vi "数据库查询.vi"() -> ()   [LabVIEW 2018]
uses:
  <vilib>/addons/_office/_exclsub.llb/font.ctl
  <vilib>/addons/database/Connection.llb/DB Tools Open Connec (String).vi
  <vilib>/addons/_office/excel.llb/Excel Easy Table (str).vi
  <vilib>/Utility/NIReport.llb/NI_report.lvclass
  <vilib>/addons/database/NI_Database_API.lvlib
  <vilib>/addons/_office/NI_ReportGenerationToolkit.lvlib
  <vilib>/Utility/NIReport.llb/Excel/NI_Excel.lvclass
panel:
  in  "Main Tab":enum32{""}(tab)
  in  "时间范围OFF":bool
  out "查询状态":string
  in  "总成码OFF":bool
  in  "刻印码":string
  in  "导出":bool
  in  "退出":bool
  in  "查询结果":i32(listbox)
  in  "查询":bool
  in  "另存为":bool
  in  "二维码OFF":bool
  in  "二维码":string
  in  "结束日期":timestamp
  in  "起始日期":timestamp
  in  "数据类型":u16(ring) items=["ALL", "Online", "Offline", "Rework"]
  in  "产品状态":u16(ring) items=["ALL", "OK", "NG"]
  # "历史数据查询"
  # "期间（过滤器）"
  # "运行"
  # "驱动数据（过滤器）"
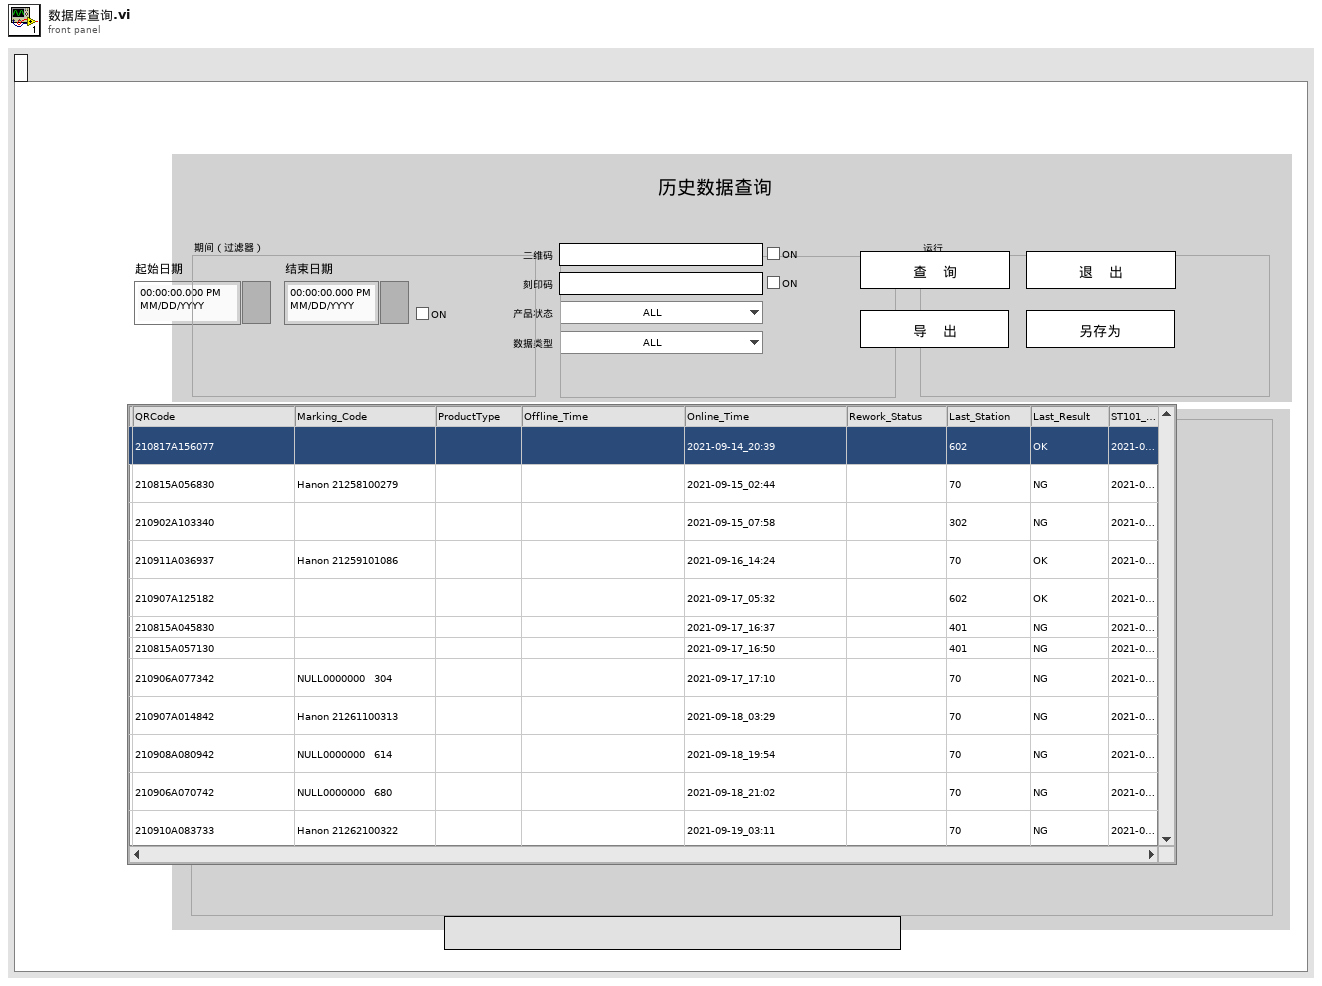
[diagram p1: front panel]
types:
  T1 = typedef "NI_ReportGenerationToolkit.lvlib/font.ctl" = cluster{"font name":string, "font size":dbl, "bold":u16, "italic":u16, "underline":u16, "strike through":u16, "font color":u32}
  T2 = enum16{"Standard Report", "HTML", "Word", "Excel"}
  T3 = enum16{"maximized", "minimized", "normal", "no change"}
  T4 = enum32{"Invalid", "Standard", "Closed", "Hidden", "Minimized", "Maximized"}
  T5 = typedef "NI_Database_API.lvlib/Conn ObjectReference.ctl" = refnum<k1>
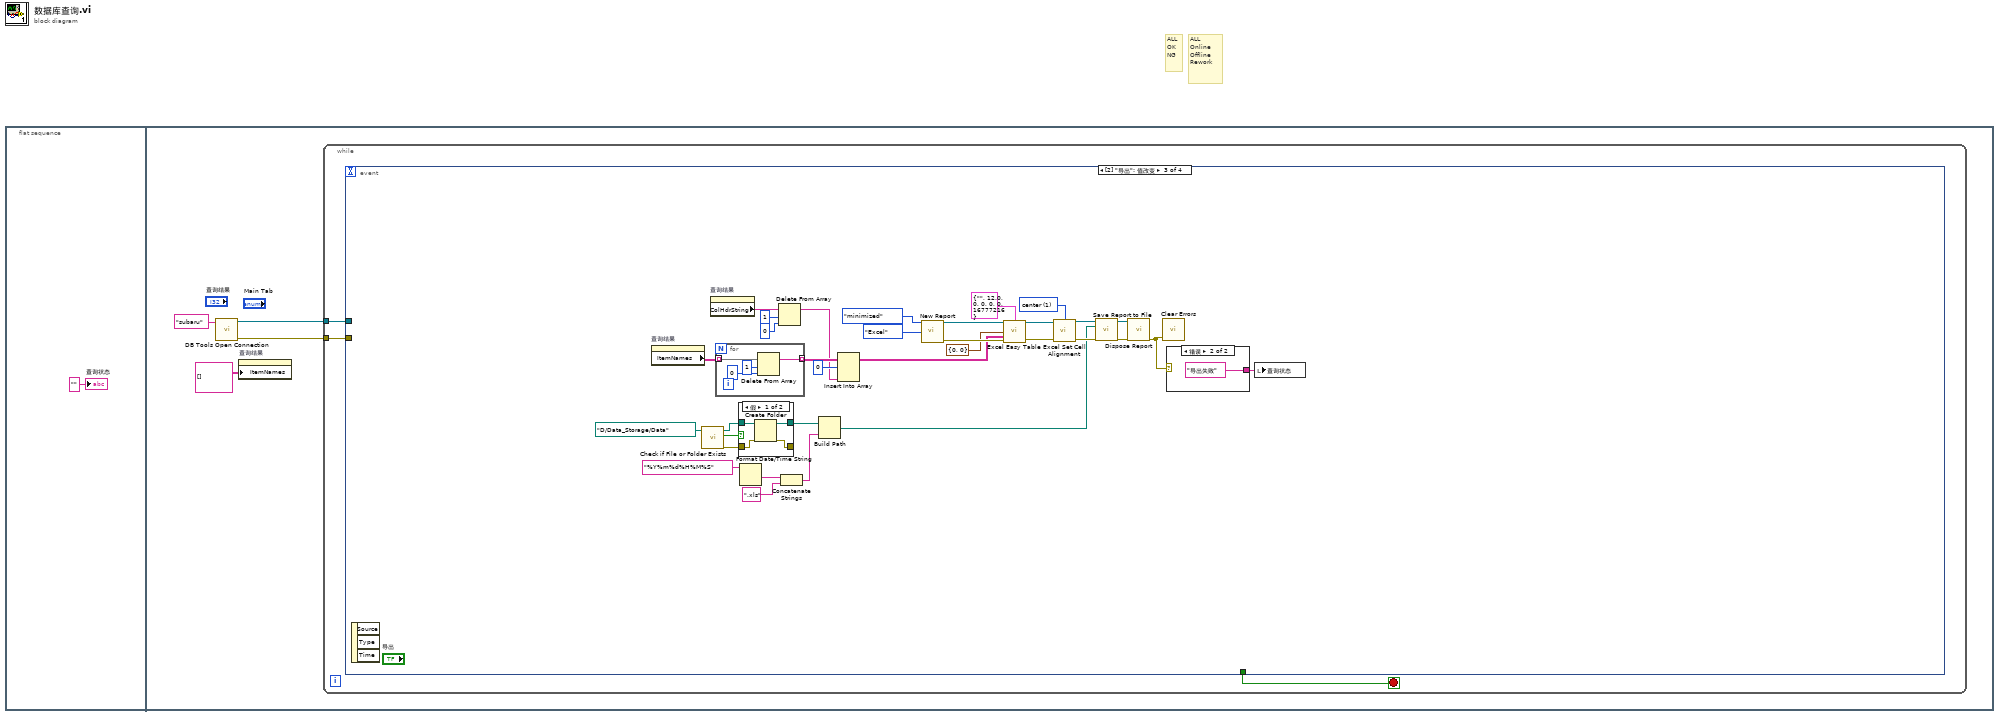
[diagram p0: block diagram]
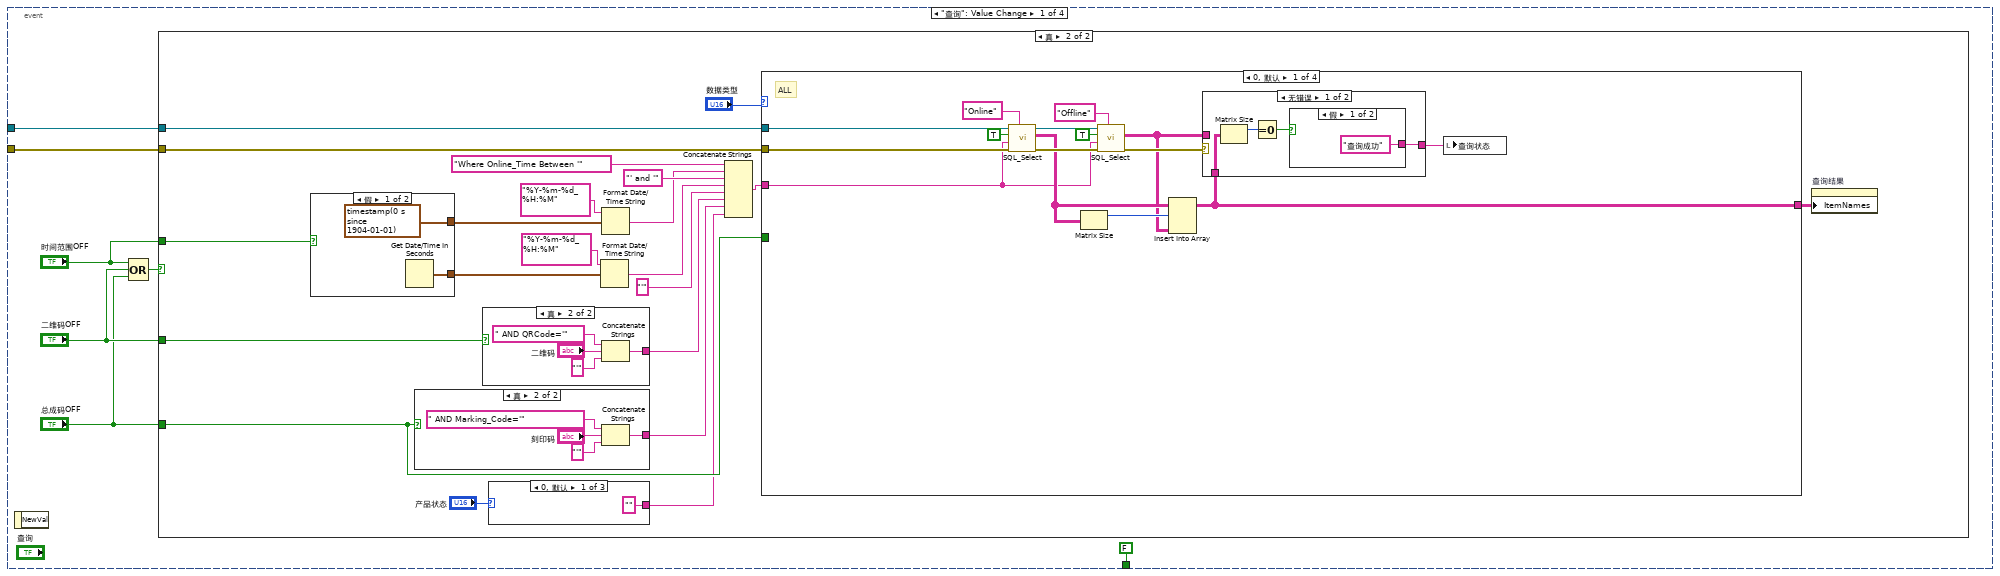
[diagram p2: hidden frame]
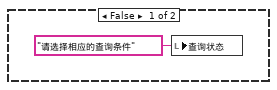
[diagram p3: hidden frame]
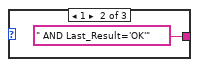
[diagram p4: hidden frame]
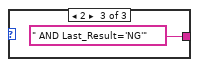
[diagram p5: hidden frame]
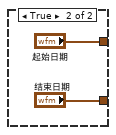
[diagram p6: hidden frame]
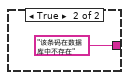
[diagram p7: hidden frame]
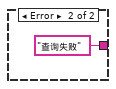
[diagram p8: hidden frame]
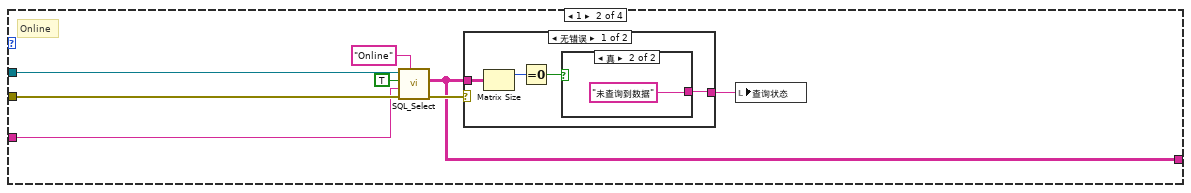
[diagram p9: hidden frame]
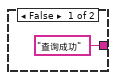
[diagram p10: hidden frame]
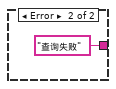
[diagram p11: hidden frame]
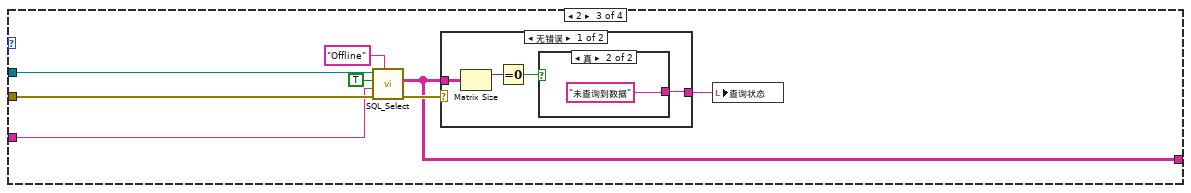
[diagram p12: hidden frame]
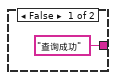
[diagram p13: hidden frame]
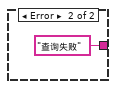
[diagram p14: hidden frame]
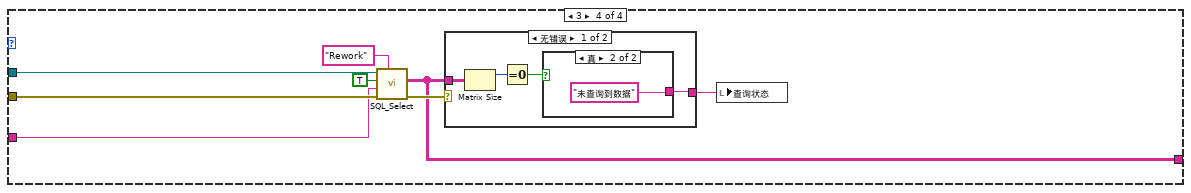
[diagram p15: hidden frame]
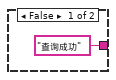
[diagram p16: hidden frame]
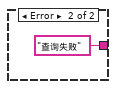
[diagram p17: hidden frame]
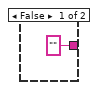
[diagram p18: hidden frame]
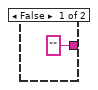
[diagram p19: hidden frame]
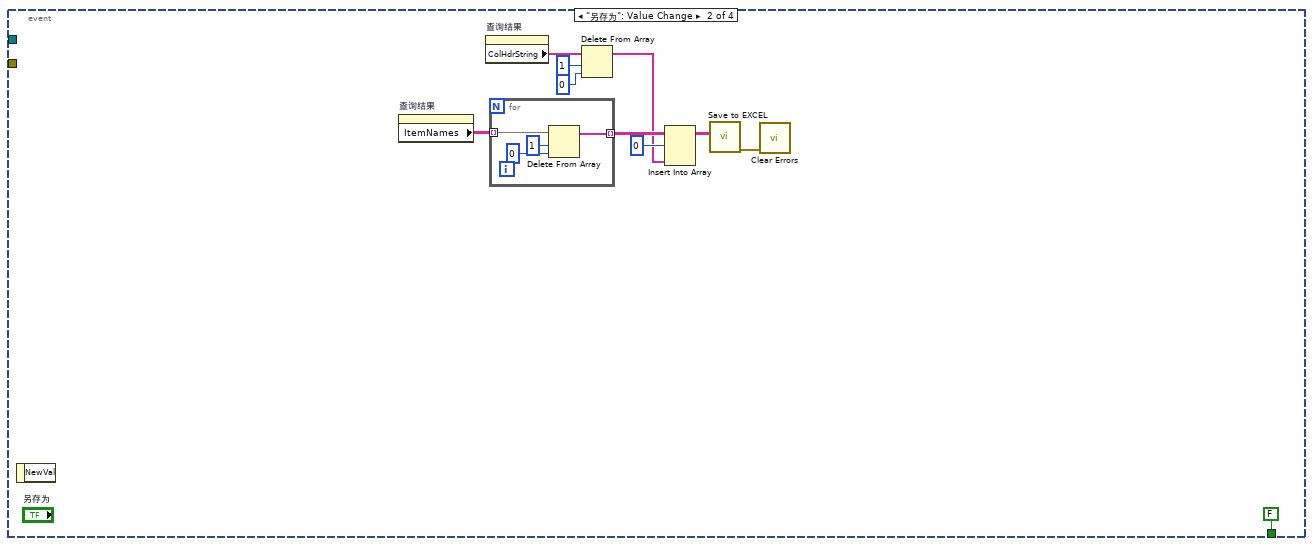
[diagram p20: hidden frame]
diagram:
  # "ALL\nOK\nNG"
  # "ALL\nOnline\nOffline\nRework"
  n1 = flat-sequence {
    frame #0 {
      "查询状态" <- "" ("查询状态")
    }
    frame #1 {
      n2 = call-poly <vilib>:"DB Tools Open Connection.vi"("connection information"="subaru") -> ("error out"=w3:errorcluster, "connection reference"=w4:T5)  [unwired: 7 in]
      n3 = property on="查询结果" class="MCListbox (严格)"("ItemNames"=string[][] [] ("项名")) -> ()  [unwired: 2 in, 2 out]
      n4 = while {
        tunnel: w4 -> [w8]
        tunnel: w3 -> [w7]
        stop <- w6 stop-if-true
        n5 = event shown="[2] \"导出\": 值改变" {
          selector: _ -> [_ _ _ _]
          dyn-events: _ -> [_ _ _ _]
          timeout: _ -> [_ _ _ _]
          tunnel: w8 -> [w15 _ _ w184]
          tunnel: w7 -> [w14 _ _ w183]
          tunnel: [FALSE ("NewVal") FALSE ("NewVal") _ w185] -> w6
          event "查询": Value Change {
            n6 = event-data() -> ()  [unwired: 1 in, 1 out]
            n7 = Compound Arithmetic op=OR("时间范围OFF", "二维码OFF", "总成码OFF") -> (w10:bool)
            n8 = case shown="真" w10 {
              tunnel: w15 -> [_ w37]
              tunnel: w14 -> [_ w36]
              tunnel: "二维码OFF" -> [_ w21]
              tunnel: "总成码OFF" -> [_ w20]
              tunnel: "时间范围OFF" -> [_ w19]
              frame False {
                n9 = local write "查询状态"("请选择相应的查询条件" ("查询状态")) -> ()
              }
              frame True {
                n10 = case shown="假" w19 {
                  tunnel: [timestamp(0 s since 1904-01-01) ("起始日期") "起始日期"] -> w32
                  tunnel: [w41 "结束日期"] -> w29
                  frame False {
                    n11 = Get Date/Time In Seconds() -> (seconds since 1Jan1904=w41:timestamp)
                  }
                  frame True {
                  }
                }
                n12 = case shown="真" w20 {
                  tunnel: ["" w114] -> w23
                  frame False {
                  }
                  frame True {
                    n13 = Concatenate Strings(" AND Marking_Code='" ("字符串"), "刻印码", "'" ("字符串")) -> (w114:string)
                  }
                }
                n14 = case shown="真" w21 {
                  tunnel: ["" w118] -> w27
                  frame False {
                  }
                  frame True {
                    n15 = Concatenate Strings(" AND QRCode='" ("字符串"), "二维码", "'" ("字符串")) -> (w118:string)
                  }
                }
                n16 = case shown="0, 默认" "产品状态" {
                  tunnel: ["" " AND Last_Result='OK'" ("字符串") " AND Last_Result='NG'" ("字符串")] -> w17
                  frame 0, Default {
                  }
                  frame 1 {
                  }
                  frame 2 {
                  }
                }
                n17 = Format Date/Time String(time format string (%c)="%Y-%m-%d_%H:%M" ("时间格式字符串(%c)"), seconds (now)=w29) -> (date/time string=w28:string)  [unwired: 1 in]
                n18 = Format Date/Time String(time format string (%c)="%Y-%m-%d_%H:%M" ("时间格式字符串(%c)"), seconds (now)=w32) -> (date/time string=w31:string)  [unwired: 1 in]
                n19 = Concatenate Strings("Where Online_Time Between '" ("查询语句"), w31, "' and '" ("字符串"), w28, "'" ("字符串"), w27, w23, w17) -> (w26:string)
                n20 = case shown="0, 默认" "数据类型" {
                  tunnel: w37 -> [w59 w70 w85 w100]
                  tunnel: w36 -> [w58 w69 w84 w99]
                  tunnel: w26 -> [w49 w68 w83 w98]
                  tunnel: [w45 w67 w82 w97] -> w25
                  tunnel: w20 -> [_ _ _ _]
                  frame 0, Default {
                    # "ALL"
                    n21 = call "SQL_Select.vi"("表名"="Online", "error in (no error)"=w58, "查询语句"=w49, "查询条件"=TRUE, "connection reference"=w59) -> ("error out"=w54:errorcluster, "数据"=w51:string[][], "connection reference out"=w53:T5)  [unwired: 4 in]
                    n22 = Matrix Size(0:w51) -> (1:w50:i32)  [unwired: 1 out]
                    n23 = call "SQL_Select.vi"("表名"="Offline", "error in (no error)"=w54, "查询语句"=w49, "查询条件"=TRUE, "connection reference"=w53) -> ("error out"=w48:errorcluster, "数据"=w46:string[][])  [unwired: 4 in, 1 out]
                    n24 = Insert Into Array(array=w51, index (row)=w50, new element=w46) -> (w45:string[][])  [unwired: 1 in]
                    n25 = case shown="无错误" w48 {
                      tunnel: [w61 "查询失败"] -> w47
                      tunnel: w46 -> [_ _]
                      tunnel: w45 -> [w60 _]
                      frame No Error {
                        n26 = Matrix Size(0:w60) -> (1:w63:i32)  [unwired: 1 out]
                        n27 = Equal To 0?(x=w63) -> (x = 0?=w62:bool)
                        n28 = case shown="假" w62 {
                          tunnel: ["查询成功" "该条码在数据库中不存在"] -> w61
                          frame False {
                          }
                          frame True {
                          }
                        }
                      }
                      frame Error {
                      }
                    }
                    n29 = local write "查询状态"(w47) -> ()
                  }
                  frame 1 {
                    # "Online"
                    n30 = call "SQL_Select.vi"("表名"="Online", "error in (no error)"=w69, "查询语句"=w68, "查询条件"=TRUE, "connection reference"=w70) -> ("error out"=w72:errorcluster, "数据"=w67:string[][])  [unwired: 4 in, 1 out]
                    n31 = case shown="无错误" w72 {
                      tunnel: [w76 "查询失败"] -> w71
                      tunnel: w67 -> [w75 _]
                      frame No Error {
                        n32 = Matrix Size(0:w75) -> (1:w78:i32)  [unwired: 1 out]
                        n33 = Equal To 0?(x=w78) -> (x = 0?=w77:bool)
                        n34 = case shown="真" w77 {
                          tunnel: ["查询成功" "未查询到数据"] -> w76
                          frame False {
                          }
                          frame True {
                          }
                        }
                      }
                      frame Error {
                      }
                    }
                    n35 = local write "查询状态"(w71) -> ()
                  }
                  frame 2 {
                    n36 = call "SQL_Select.vi"("表名"="Offline", "error in (no error)"=w84, "查询语句"=w83, "查询条件"=TRUE, "connection reference"=w85) -> ("error out"=w87:errorcluster, "数据"=w82:string[][])  [unwired: 4 in, 1 out]
                    n37 = case shown="无错误" w87 {
                      tunnel: [w91 "查询失败"] -> w86
                      tunnel: w82 -> [w90 _]
                      frame No Error {
                        n38 = Matrix Size(0:w90) -> (1:w93:i32)  [unwired: 1 out]
                        n39 = Equal To 0?(x=w93) -> (x = 0?=w92:bool)
                        n40 = case shown="真" w92 {
                          tunnel: ["查询成功" "未查询到数据"] -> w91
                          frame False {
                          }
                          frame True {
                          }
                        }
                      }
                      frame Error {
                      }
                    }
                    n41 = local write "查询状态"(w86) -> ()
                  }
                  frame 3 {
                    n42 = call "SQL_Select.vi"("表名"="Rework", "error in (no error)"=w99, "查询语句"=w98, "查询条件"=TRUE, "connection reference"=w100) -> ("error out"=w104:errorcluster, "数据"=w97:string[][])  [unwired: 4 in, 1 out]
                    n43 = case shown="无错误" w104 {
                      tunnel: [w106 "查询失败"] -> w103
                      tunnel: w97 -> [w105 _]
                      frame No Error {
                        n44 = Matrix Size(0:w105) -> (1:w108:i32)  [unwired: 1 out]
                        n45 = Equal To 0?(x=w108) -> (x = 0?=w107:bool)
                        n46 = case shown="真" w107 {
                          tunnel: ["查询成功" "未查询到数据"] -> w106
                          frame False {
                          }
                          frame True {
                          }
                        }
                      }
                      frame Error {
                      }
                    }
                    n47 = local write "查询状态"(w103) -> ()
                  }
                }
                n48 = property on="查询结果" class="MCListbox (严格)"("ItemNames"=w25) -> ()  [unwired: 2 in, 2 out]
              }
            }
          }
          event "另存为": Value Change {
            n49 = event-data() -> ()  [unwired: 1 in, 1 out]
            n50 = property on="查询结果" class="MCListbox (严格)"() -> ("ItemNames"=w127:string[][])  [unwired: 2 in, 2 out]
            n51 = property on="查询结果" class="MCListbox (严格)"() -> ("ColHdrString"=w130:string[])  [unwired: 2 in, 2 out]
            n52 = for {
              tunnel: w127 -> [w135] mode=indexing
              tunnel: [w132] -> w125 mode=indexing
              n53 = Delete From Array(array=w135, length=1 ("长度"), index=0 ("索引")) -> (array with subset deleted=w132:string[])  [unwired: 1 out]
            }
            n54 = Delete From Array(array=w130, length=1 ("长度"), index=0 ("索引")) -> (array with subset deleted=w124:string[])  [unwired: 1 out]
            n55 = Insert Into Array(array=w125, index (row)=0 ("索引"), new element=w124) -> (w123:string[][])  [unwired: 1 in]
            n56 = call "Save to EXCEL.vi"("text data"=w123) -> ("error out"=w122:errorcluster)  [unwired: 10 in]
            n57 = call <vilib>:"Clear Errors.vi"("error in (no error)"=w122) -> ()  [unwired: 5 in, 2 out]
          }
          event "导出": Value Change {
            w158 = 1 items=["left", "center", "right"] ("horizontal alignment (left)")
            n58 = event-data() -> ()  [unwired: 1 in, 3 out]
            n59 = property on="查询结果" class="MCListbox (严格)"() -> ("ItemNames"=w165:string[][])  [unwired: 2 in, 2 out]
            n60 = call <vilib>:"Check if File or Folder Exists.vi"("path"=path "D:/Data_Storage/Data" ("文件路径（使用对话框）")) -> ("error out"=w144:errorcluster, "file or folder exists?"=w146:bool, "dup path"=w145:path)  [unwired: 8 in]
            n61 = property on="查询结果" class="MCListbox (严格)"() -> ("ColHdrString"=w168:string[])  [unwired: 2 in, 2 out]
            n62 = for {
              tunnel: w165 -> [w180] mode=indexing
              tunnel: [w177] -> w163 mode=indexing
              n63 = Delete From Array(array=w180, length=1 ("长度"), index=0 ("索引")) -> (array with subset deleted=w177:string[])  [unwired: 1 out]
            }
            n64 = case shown="假" w146 {
              tunnel: w145 -> [w174 w176]
              tunnel: [w173 w176] -> w140
              tunnel: w144 -> [w172 w175]
              tunnel: [w171 w175] -> _
              frame False {
                n65 = Create Folder(path (use dialog)=w174, error in=w172) -> (created path=w173:path, error out=w171:errorcluster)  [unwired: 1 in, 1 out]
              }
              frame True {
              }
            }
            n66 = Format Date/Time String(time format string (%c)="%Y%m%d%H%M%S" ("时间格式字符串(%c)")) -> (date/time string=w142:string)  [unwired: 2 in]
            n67 = Delete From Array(array=w168, length=1 ("长度"), index=0 ("索引")) -> (array with subset deleted=w162:string[])  [unwired: 1 out]
            n68 = Concatenate Strings(w142, ".xls" ("字符串")) -> (w139:string)
            n69 = Build Path(base path=w140, name or relative path=w139) -> (appended path=w138:path)
            n70 = Insert Into Array(array=w163, index (row)=0 ("索引"), new element=w162) -> (w148:string[][])  [unwired: 1 in]
            n71 = call <vilib>:"New Report.vi"("window state (normal)"=T3."minimized", "report type"=T2."Excel") -> ("report out"=w154:refnum<class "NI_report.lvclass">, "error out"=w155:errorcluster)  [unwired: 12 in]
            n72 = call-poly <vilib>:"Excel Easy Table.vi"("report in"=w154, "font"=T1 {"font name"="", "font size"=12.0, "bold"=0, "italic"=0, "underline"=0, "strike through"=0, "font color"=16777216}, "start (0, 0)"=cluster{"row":i32, "column":i32} {"row"=0, "column"=0}, "text data"=w148, "error in (no error)"=w155) -> ("report out"=w156:refnum<class "NI_report.lvclass">, "error out"=w157:errorcluster)  [unwired: 6 in, 3 out]
            n73 = call <vilib>:"Excel Set Cell Alignment.vi"("report in"=w156, "horizontal alignment (left)"=w158, "error in (no error)"=w157) -> ("report out"=w149:refnum<class "NI_report.lvclass">, "error out"=w152:errorcluster)  [unwired: 11 in]
            n74 = call-dynamic "Save Report to File.vi"("report in"=w149, "report file path"=w138, "error in (no error)"=w152) -> ("report out"=w150:refnum<class "NI_report.lvclass">, "error out"=w151:errorcluster)  [unwired: 11 in]
            n75 = call-dynamic "Dispose Report.vi"("report in"=w150, "error in (no error)"=w151) -> ("error out"=w137:errorcluster)  [unwired: 13 in]
            n76 = call <vilib>:"Clear Errors.vi"("error in (no error)"=w137) -> ()  [unwired: 5 in, 2 out]
            n77 = case shown="错误" w137 {
              tunnel: ["导出成功" "导出失败"] -> w136
              frame No Error {
              }
              frame Error {
              }
            }
            n78 = local write "查询状态"(w136) -> ()
          }
          event "退出": Value Change {
            n79 = event-data() -> ("NewVal"=w185:bool)  [unwired: 1 in]
            n80 = call <vilib>:"DB Tools Close Connection.vi"("error in (no error)"=w183, "connection reference"=w184) -> ()  [unwired: 5 in, 1 out]
            n81 = control-ref of="本VI"() -> (w182:refnum<vi>)
            n82 = property class="VI"(reference=w182, "FP.State"=T4."Closed" ("前面板窗口:状态")) -> ()  [unwired: 1 in, 2 out]
          }
        }
      }
    }
  }
